vi "Deserialize32.vi"(11 "U32 input":u32) -> (3 "30bit output":bool[](array[boolean]))   [LabVIEW 2012]
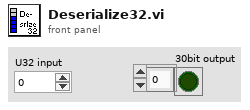
[diagram p1: front panel]
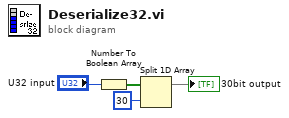
[diagram p0: block diagram]
diagram:
  n1 = Number To Boolean Array(number="U32 input") -> (Boolean array=w3:bool[])
  n2 = Split 1D Array(array=w3, index=30) -> (first subarray=→"30bit output":bool[])  [unwired: 1 out]
